vi "Decode Display.vi"(7 "Segment Pattern":string[](array[string]), 11 "Display":string[](array[string])) -> (3 "Value on Display":i64)   [LabVIEW 2021]
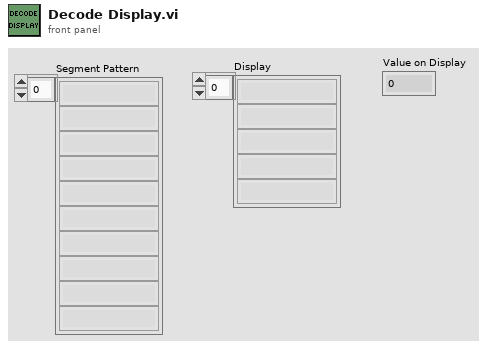
[diagram p1: front panel]
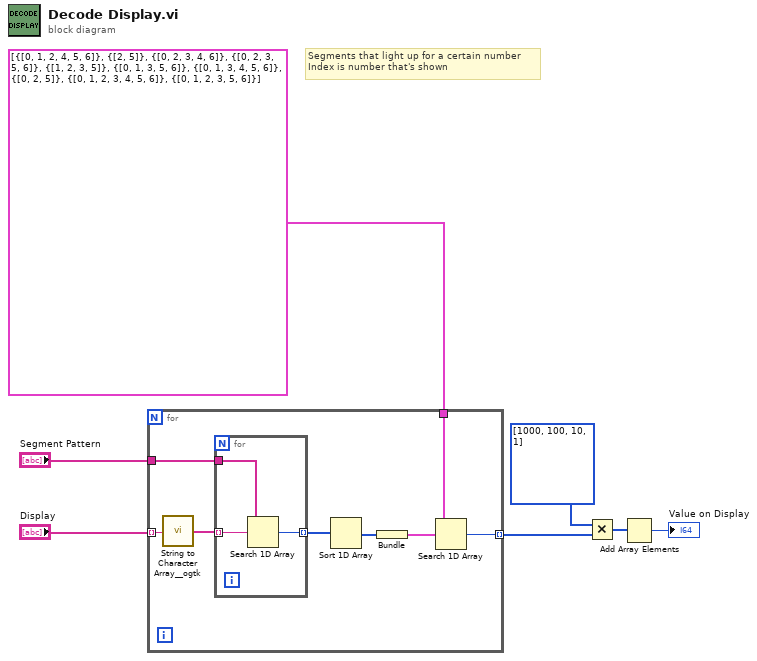
[diagram p0: block diagram]
diagram:
  # "Segments that light up for a certain number\nIndex is number that's shown"
  n1 = for {
    tunnel: "Display" -> [w15] mode=indexing
    tunnel: "Segment Pattern" -> [w14]
    tunnel: cluster{i32[]}[] [{[0, 1, 2, 4, 5, 6]}, {[2, 5]}, {[0, 2, 3, 4, 6]}, {[0, 2, 3, 5, 6]}, {[1, 2, 3, 5]}, {[0, 1, 3, 5, 6]}, {[0, 1, 3, 4, 5, 6]}, {[0, 2, 5]}, {[0, 1, 2, 3, 4, 5, 6]}, {[0, 1, 2, 3, 5, 6]}] -> [w10]
    tunnel: [w9] -> w4 mode=indexing
    n2 = call <userlib>:"String to Character Array__ogtk.vi"("Input String"=w15) -> ("Character Array"=w8:string[])
    n3 = for {
      tunnel: w14 -> [w18]
      tunnel: w8 -> [w17] mode=indexing
      tunnel: [w16] -> w13 mode=indexing
      n4 = Search 1D Array(1D array=w18, element=w17) -> (index of element=w16:i32)  [unwired: 1 in]
    }
    n5 = Sort 1D Array(array=w13) -> (sorted array=w12:i32[])
    n6 = Bundle(w12) -> (w11:cluster{i32[]})  [unwired: 1 in]
    n7 = Search 1D Array(1D array=w10, element=w11) -> (index of element=w9:i32)  [unwired: 1 in]
  }
  n8 = Multiply(x=i64[] [1000, 100, 10, 1], y=w4) -> (x*y=w3:i64[])
  n9 = Add Array Elements(numeric array=w3) -> (sum=→"Value on Display":i64)
